vi "followMotionProfile.vi"(9 "Constants":T1={"kV"=0.00542, "kA"=0.0008, "Velocity PID"={"P"=1.0, "I"=0.01, "D"=0.0}, "Position PID"={"P"=1.0, "I"=0.01, "D"=0.0}}, 10 "Feedback":cluster{"accel":dbl, "vel":dbl, "pos":dbl}, 11 "Target":cluster{"accel":dbl, "vel":dbl, "pos":dbl}) -> (3 "Duty Cycle":dbl)   [LabVIEW 2016]
uses:
  <vilib>/addons/control/pid/pid.llb/PID (DBL).vi
  <vilib>/addons/control/pid/NI_PID_pid.lvlib
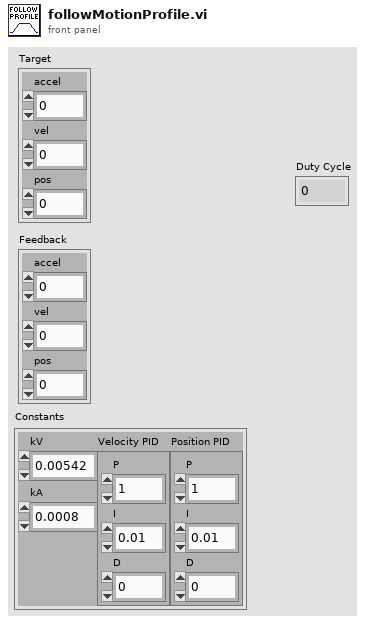
[diagram p1: front panel]
types:
  T1 = cluster{"kV":dbl, "kA":dbl, "Velocity PID":cluster{"P":dbl, "I":dbl, "D":dbl}, "Position PID":cluster{"P":dbl, "I":dbl, "D":dbl}}
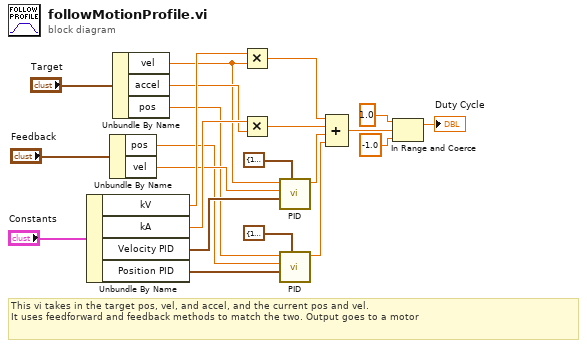
[diagram p0: block diagram]
diagram:
  # "This vi takes in the target pos, vel, and accel, and the current pos and vel.\nIt uses feedforward and feedback methods to match the two. Output goes to a motor"
  n1 = Unbundle By Name("Constants") -> ("kV"=w12:dbl, "kA"=w11:dbl, "Velocity PID"=w9:cluster{"P":dbl, "I":dbl, "D":dbl}, "Position PID"=w2:cluster{"P":dbl, "I":dbl, "D":dbl})
  n2 = Unbundle By Name("Feedback") -> ("pos"=w3:dbl, "vel"=w7:dbl)
  n3 = Unbundle By Name("Target") -> ("vel"=w8:dbl, "accel"=w10:dbl, "pos"=w4:dbl)
  n4 = Multiply(x=w12, y=w8) -> (x*y=w20:dbl)
  n5 = Multiply(x=w11, y=w10) -> (x*y=w21:dbl)
  n6 = call-poly <vilib>:"PID.vi"("output range"=cluster{"output high":dbl, "output low":dbl} {"output high"=1.0, "output low"=-1.0}, "PID gains"=w9, "process variable"=w7, "setpoint"=w8) -> ("output"=w6:dbl)  [unwired: 6 in, 1 out]
  n7 = call-poly <vilib>:"PID.vi"("output range"=cluster{"output high":dbl, "output low":dbl} {"output high"=1.0, "output low"=-1.0}, "PID gains"=w2, "process variable"=w3, "setpoint"=w4) -> ("output"=w1:dbl)  [unwired: 6 in, 1 out]
  n8 = Compound Arithmetic op=ADD(w20, w21, w6, w1) -> (w19:dbl)
  n9 = In Range and Coerce(upper limit=1.0, x=w19, lower limit=-1.0) -> (coerced(x)=→"Duty Cycle":dbl)  [unwired: 1 out]
